vi "TDMSToTXTFileDataManager.vi"(4 "entrée d'erreur":errorcluster, 5 "Info(analog acq,wave,Quali,hexap...)":string, 6 "FichierTDMSOrigine":path, 7 "NomProj":string) -> (0 "sortie d'erreur":errorcluster, 2 "chemin complet":path, 3 "NomProjOUT":string)   [LabVIEW 2017]
uses:
  DefDeType/WhichPath.ctl
  <vilib>/Waveform/WDTOps.llb/WDT Index Channel DBL.vi
  <vilib>/Waveform/WDTOps.llb/WDT Get Waveform Time Array DBL.vi
panel:
  out "Tableau":dbl[](array[numeric])
  out "Units":string[](array[string])
  out "Waveforms":waveform(dbl)[](graph)
  out "Noms des voies":string[](array[string])
  out "Y":dbl[][](array[numeric])
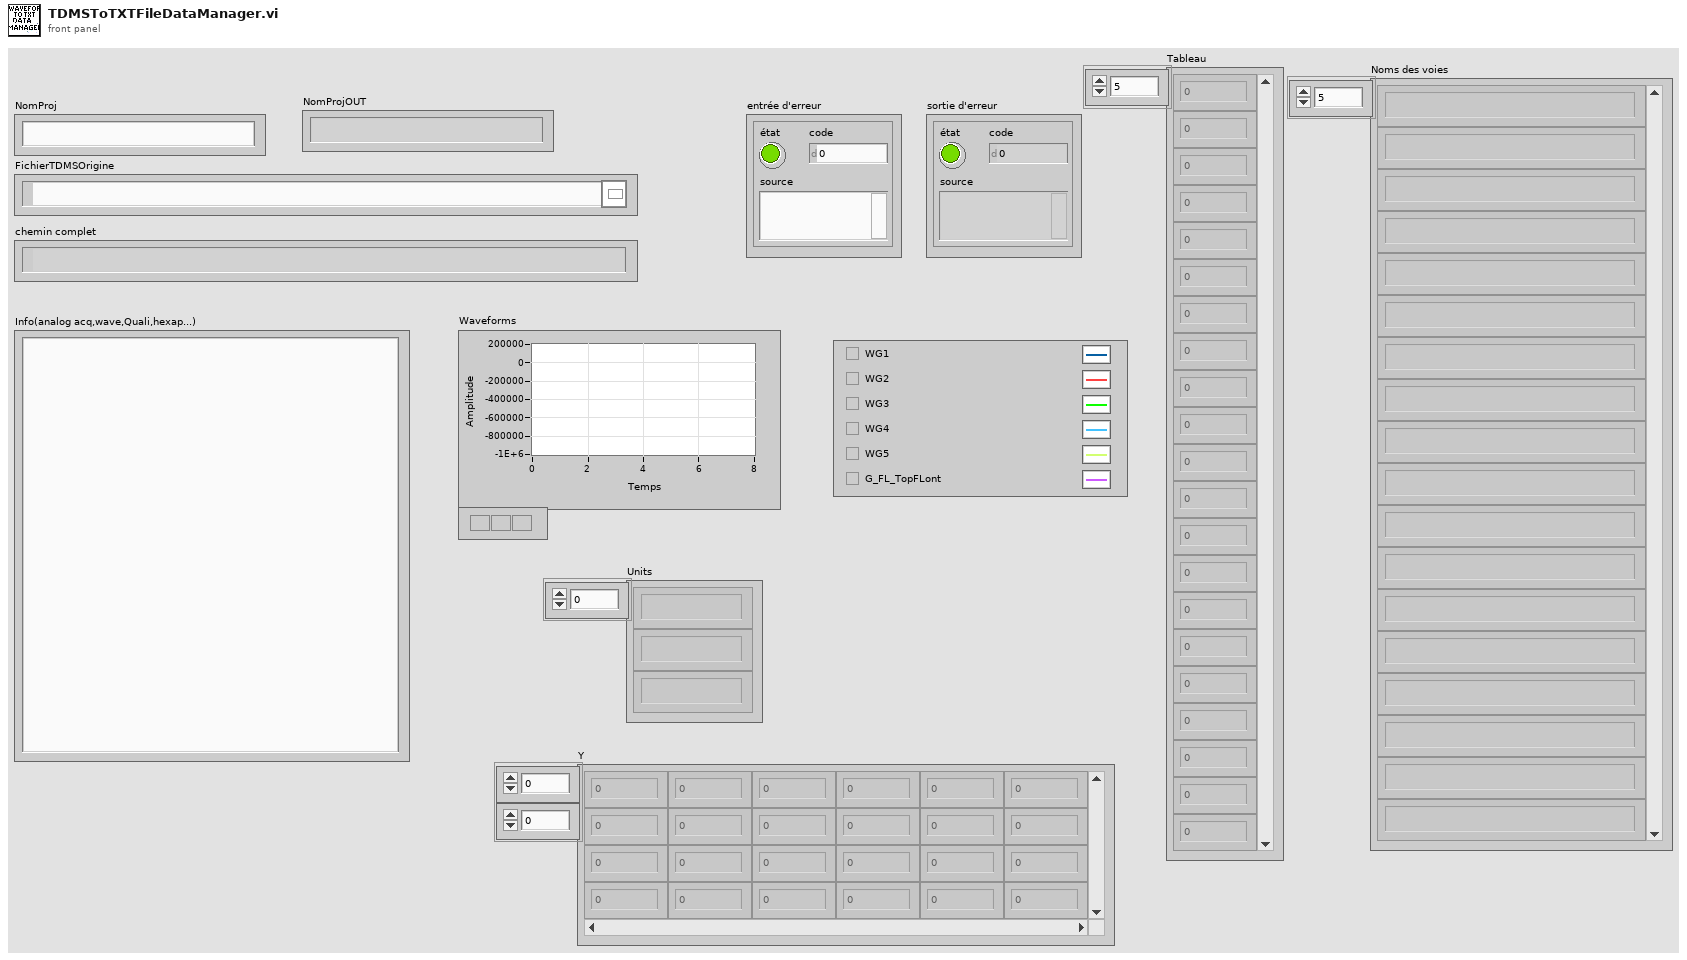
[diagram p1: front panel]
types:
  T1 = typedef "WhichPath.ctl" = enum16{"DossierProjet", "Config", "Meas", "MeasPCI", "MeasCRIO1", "MeasCRIO2", "MeasQualisys", "MeasHBM", "MeasTDMS", "Fig", "Res"}
  T2 = enum16{"open", "replace", "create", "open or create", "replace or create", "replace or create with confirmation"}
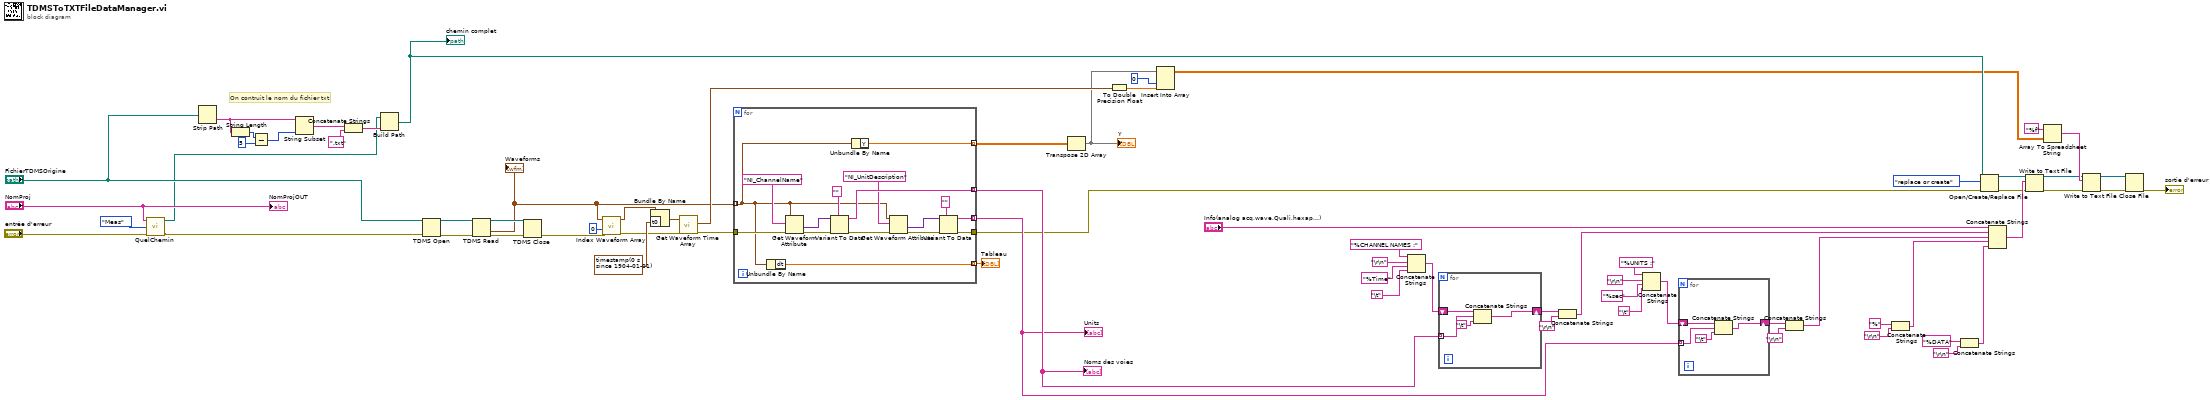
[diagram p0: block diagram]
diagram:
  # "On contruit le nom du fichier txt"
  n1 = call "QuelChemin.vi"("Entrée d'erreur"="entrée d'erreur", "WhichPath?"=WhichPath."Meas", "NomProjet"="NomProj") -> ("Sortie d'erreur"=w3:errorcluster, "SurDisqueLocal"=w2:path)  [unwired: 1 out]
  n2 = Strip Path(path="FichierTDMSOrigine") -> (name=w44:string)  [unwired: 1 out]
  n3 = String Length(string=w44) -> (length=w43:i32)
  n4 = Subtract(x=w43, y=5) -> (x-y=w46:i32)
  n5 = String Subset(string=w44, length (rest)=w46) -> (substring=w45:string)  [unwired: 1 in]
  n6 = Concatenate Strings(w45, ".txt" ("chaîne")) -> (w48:string)
  n7 = Build Path(base path=w2, name or relative path=w48) -> (appended path=w50:path)
  "chemin complet" <- w50
  n8 = TDMS Open(8:w3, 11:"FichierTDMSOrigine") -> (0:w41:errorcluster, 3:w42:refnum<k34>)  [unwired: 5 in]
  n9 = TDMS Read(0:w42, 11:w41) -> (4:w52:refnum<k34>, 10:w13:waveform(dbl)[], 15:w53:errorcluster)  [unwired: 6 in, 3 out]
  "Waveforms" <- w13
  n10 = TDMS Close(8:w53, 11:w52) -> (0:w20:errorcluster)  [unwired: 1 out]
  n11 = call-poly <vilib>:"Index Waveform Array.vi"("error in (no error)"=w20, "index"=0, "waveform array"=w13) -> ("error out"=w21:errorcluster, "waveform"=w12:waveform(dbl))  [unwired: 7 in]
  n12 = Bundle By Name(cluster=w12, "t0"=timestamp(0 s since 1904-01-01)) -> (w23:waveform(dbl))
  n13 = call-poly <vilib>:"Get Waveform Time Array.vi"("error in (no error)"=w21, "waveform in"=w23) -> ("error out"=w19:errorcluster, "X array"=w16:timestamp[])  [unwired: 8 in]
  n14 = for {
    tunnel: w13 -> [w72] mode=indexing
    tunnel: [w86] -> w70 mode=indexing
    tunnel: [w74] -> w9
    tunnel: w19 -> [w76]
    tunnel: [w81] -> w28 mode=indexing
    tunnel: [w73] -> w27 mode=indexing
    tunnel: [w71] -> w1 mode=indexing
    n15 = Unbundle By Name(w72) -> ("dt"=w71:dbl)
    n16 = Get Waveform Attribute(4:w76, 6:"NI_ChannelName" ("nom"), 7:w72) -> (0:w85:errorcluster, 1:w83:variant)  [unwired: 1 in, 2 out]
    n17 = Variant To Data(error in=w85, type="" ("nom"), Variant=w83) -> (data=w81:string, error out=w75:errorcluster)
    n18 = Unbundle By Name(w72) -> ("Y"=w86:dbl[])
    n19 = Get Waveform Attribute(4:w75, 6:"NI_UnitDescription" ("nom"), 7:w72) -> (0:w77:errorcluster, 1:w78:variant)  [unwired: 1 in, 2 out]
    n20 = Variant To Data(error in=w77, type="" ("nom"), Variant=w78) -> (data=w73:string, error out=w74:errorcluster)
  }
  "Noms des voies" <- w28
  "Units" <- w27
  "Tableau" <- w1
  n21 = Transpose 2D Array(2D array=w70) -> (transposed array=w15:dbl[][])
  "Y" <- w15
  n22 = To Double Precision Float(number=w16) -> (double precision float=w17:dbl[])
  n23 = Insert Into Array(array=w15, index (col)=0 ("indice désactivé (col)"), new element=w17) -> (w14:dbl[][])  [unwired: 1 in]
  n24 = Concatenate Strings("%CHANNEL NAMES :" ("chaîne"), "\r\n", "%Time" ("chaîne"), "\t") -> (w36:string)
  n25 = for {
    tunnel: w28 -> [w88] mode=indexing
    shift-right: [w90] -> w67
    shift-left: w36 -> [w89]
    n26 = Concatenate Strings(w89, w88, "\t") -> (w90:string)
  }
  n27 = Concatenate Strings(w67, "\r\n") -> (w11:string)
  n28 = Concatenate Strings("%UNITS :" ("chaîne"), "\r\n", "%sec" ("chaîne"), "\t") -> (w32:string)
  n29 = for {
    tunnel: w27 -> [w92] mode=indexing
    shift-right: [w94] -> w55
    shift-left: w32 -> [w93]
    n30 = Concatenate Strings(w93, w92, "\t") -> (w94:string)
  }
  n31 = Concatenate Strings(w55, "\r\n") -> (w10:string)
  n32 = Concatenate Strings("%" ("chaîne"), "\r\n") -> (w40:string)
  n33 = Concatenate Strings("%DATA" ("chaîne"), "\r\n") -> (w29:string)
  n34 = Open/Create/Replace File(file path (use dialog)=w50, error in=w9, operation (0:open)=T2."replace or create" ("opération (0 : open)")) -> (refnum out=w63:refnum<file>, error out=w62:errorcluster)  [unwired: 3 in, 1 out]
  n35 = Concatenate Strings("Info(analog acq,wave,Quali,hexap...)", w11, w10, w40, w29) -> (w64:string)
  n36 = Write to Text File(file (use dialog)=w63, text=w64, error in=w62) -> (refnum out=w57:refnum<file>, error out=w61:errorcluster)  [unwired: 1 in, 1 out]
  n37 = Array To Spreadsheet String(array=w14, 3:"%f" ("chaîne de format")) -> (spreadsheet string=w58:string)  [unwired: 1 in]
  n38 = Write to Text File(file (use dialog)=w57, text=w58, error in=w61) -> (refnum out=w56:refnum<file>, error out=w60:errorcluster)  [unwired: 1 in, 1 out]
  n39 = Close File(refnum=w56, error in=w60) -> (error out=→"sortie d'erreur":errorcluster)  [unwired: 1 out]
  "NomProjOUT" <- "NomProj"
